vi "xyPlot.vi"(6 "fill?(F)":bool=TRUE, 7 "radius":i16=5, 9 "Array In":dbl[][](array[numeric]), 11 "new picture in":picture) -> (1 "Array Out":dbl[][](array[numeric]), 3 "new picture out":picture)   [LabVIEW 2020]
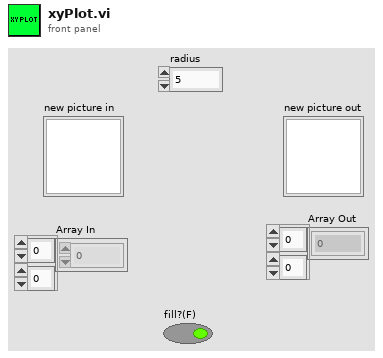
[diagram p1: front panel]
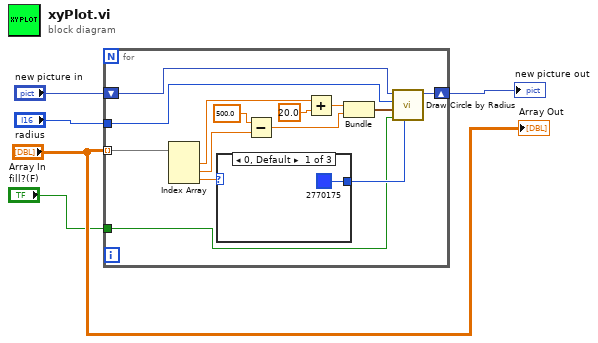
[diagram p0: block diagram]
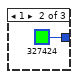
[diagram p2: hidden frame]
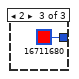
[diagram p3: hidden frame]
diagram:
  n1 = for {
    shift-right: [w13] -> w4
    shift-left: "new picture in" -> [w19]
    tunnel: "Array In" -> [w12] mode=indexing
    tunnel: "radius" -> [w7]
    tunnel: "fill?(F)" -> [w6]
    n2 = Index Array(array=w12) -> (element #1=w11:dbl, element #2=w10:dbl, element #3=w9:dbl)  [unwired: 3 in]
    n3 = case shown="0, Default" w9 {
      tunnel: [u32 2770175 ("color(black)") u32 327424 ("color(black)") u32 16711680 ("color(black)")] -> w8
      frame 0, Default {
      }
      frame 1 {
      }
      frame 2 {
      }
    }
    n4 = Subtract(x=500.0, y=w10) -> (x-y=w15:dbl)
    n5 = Add(x=w11, y=20.0) -> (x+y=w18:dbl)
    n6 = Bundle(w18, w15) -> (w16:cluster{dbl, dbl})  [unwired: 1 in]
    n7 = call <vilib>:"Draw Circle by Radius.vi"("color(black)"=w8, "fill?(F)"=w6, "pixel center"=w16, "radius"=w7, "picture"=w19) -> ("new picture"=w13:picture)  [unwired: 6 in]
  }
  "new picture out" <- w4
  "Array Out" <- "Array In"
